vi "ODMR sweep set MW control.vi"(8 "Save?":bool, 9 "file path (dialog if empty)":path=path "C:/Users/Ouyang Group/Documents/Data/5-13-15/ND Au 686 ODMR sweep 1", 10 "Freq Sweep Cluster":T1={"GPIB address 2"="19", "resolution (10 Hz:2) 2"=2, "band (1-26.5:2) 2"=2, "Freq max"=3300000000.0, "Start Freq"=5.5, "freq Step"=0.02, "rate"=100.0, "samples per channel"=500} {"rate" format="%0.2f"; "resolution (10 Hz:2) 2" items=["0.1 Hz", "1 Hz", "10 Hz", "100 Hz", "1 KHz", "10 KHz", "100 KHz", "1 MHz", "10 MHz", "100 MHz", "1 GHz"]}, 11 "Dot Tracking Cluster":T2={"RS232 settings"={"Portnumber"=6, "Baudrate"=5}, "X Parameters"={"Number of X Steps"=200, "Max X (V)"=2.0, "Min X (V)"=-2.0}, "Y Parameters"={"Number of Y Steps"=200, "Max Y (V)"=2.0, "Min Y (V)"=-2.0}, "X Pos"=97.0, "Y Pos"=112.0, "Z Pos"=52.78, "Tracking interval"=150.0} {"RS232 settings"."Portnumber" items=["COM1", "COM2", "COM3", "COM4", "COM5", "COM6", "COM7", "COM8", "COM9", "COM10", "COM11", "COM12", "COM13", "COM14", "COM15", "COM16", "COM17", "COM18", "COM19", "COM20", "COM21", "COM22", "COM23", "COM24", "COM25", "COM26", "COM27", "COM28", "COM29", "COM30"]; "RS232 settings"."Baudrate" items=["9600", "14400", "19200", "38400", "57600", "115200"]}) -> (0 "Z Position":dbl=31.0, 1 "Y Position":dbl=62.0, 2 "X Position":dbl=97.0, 3 "XY Graph":cluster{"Y":dbl[], "Y":dbl[]}[](graph), 4 "appended array":ext[][](array[numeric]))   [LabVIEW 2012]
uses:
  <vilib>/DAQmx/read.llb/DAQmx Read (Counter 1D DBL 1Chan NSamp).vi
  <vilib>/DAQmx/create/channels.llb/DAQmx Create Channel (CI-Count Edges).vi
  <vilib>/DAQmx/configure/timing.llb/DAQmx Timing (Sample Clock).vi
  <vilib>/DAQmx/miscellaneous.llb/DAQmx Fill In Error Info.vi
  <vilib>/Utility/file.llb/Write To Spreadsheet File (DBL).vi
  <resource>/objmgr/daqmx.rc
panel:
  out "power compensated":ext
  out "freq":dbl
  in  "stop":bool
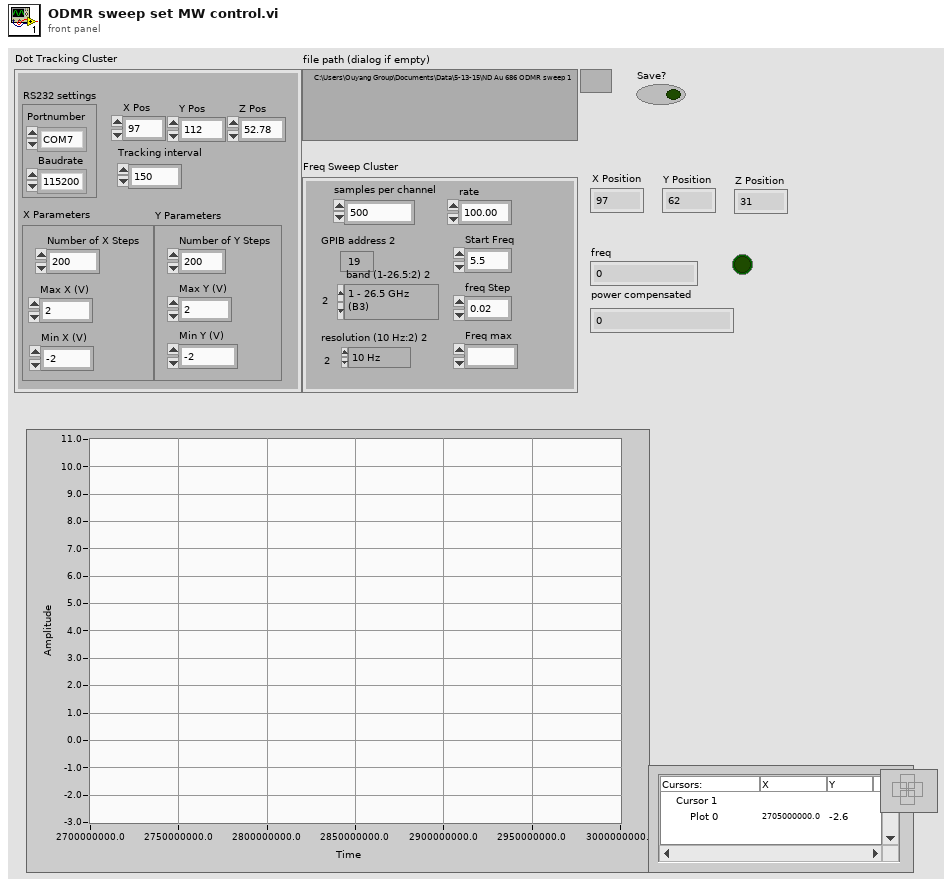
[diagram p1: front panel]
types:
  T1 = cluster{"GPIB address 2":string, "resolution (10 Hz:2) 2":i32, "band (1-26.5:2) 2":i32, "Freq max":ext, "Start Freq":dbl, "freq Step":dbl, "rate":dbl, "samples per channel":i32}
  T2 = cluster{"RS232 settings":cluster{"Portnumber":i32, "Baudrate":u16}, "X Parameters":cluster{"Number of X Steps":i32, "Max X (V)":dbl, "Min X (V)":dbl}, "Y Parameters":cluster{"Number of Y Steps":i32, "Max Y (V)":dbl, "Min Y (V)":dbl}, "X Pos":dbl, "Y Pos":dbl, "Z Pos":dbl, "Tracking interval":dbl}
  T3 = cluster{"Number of X Steps":i32, "Max X (V)":dbl, "Min X (V)":dbl}
  T4 = cluster{"Number of Y Steps":i32, "Max Y (V)":dbl, "Min Y (V)":dbl}
  T5 = cluster{"source lock":bool, "lock frequency (Hz)":ext, "coarse tune":bool}
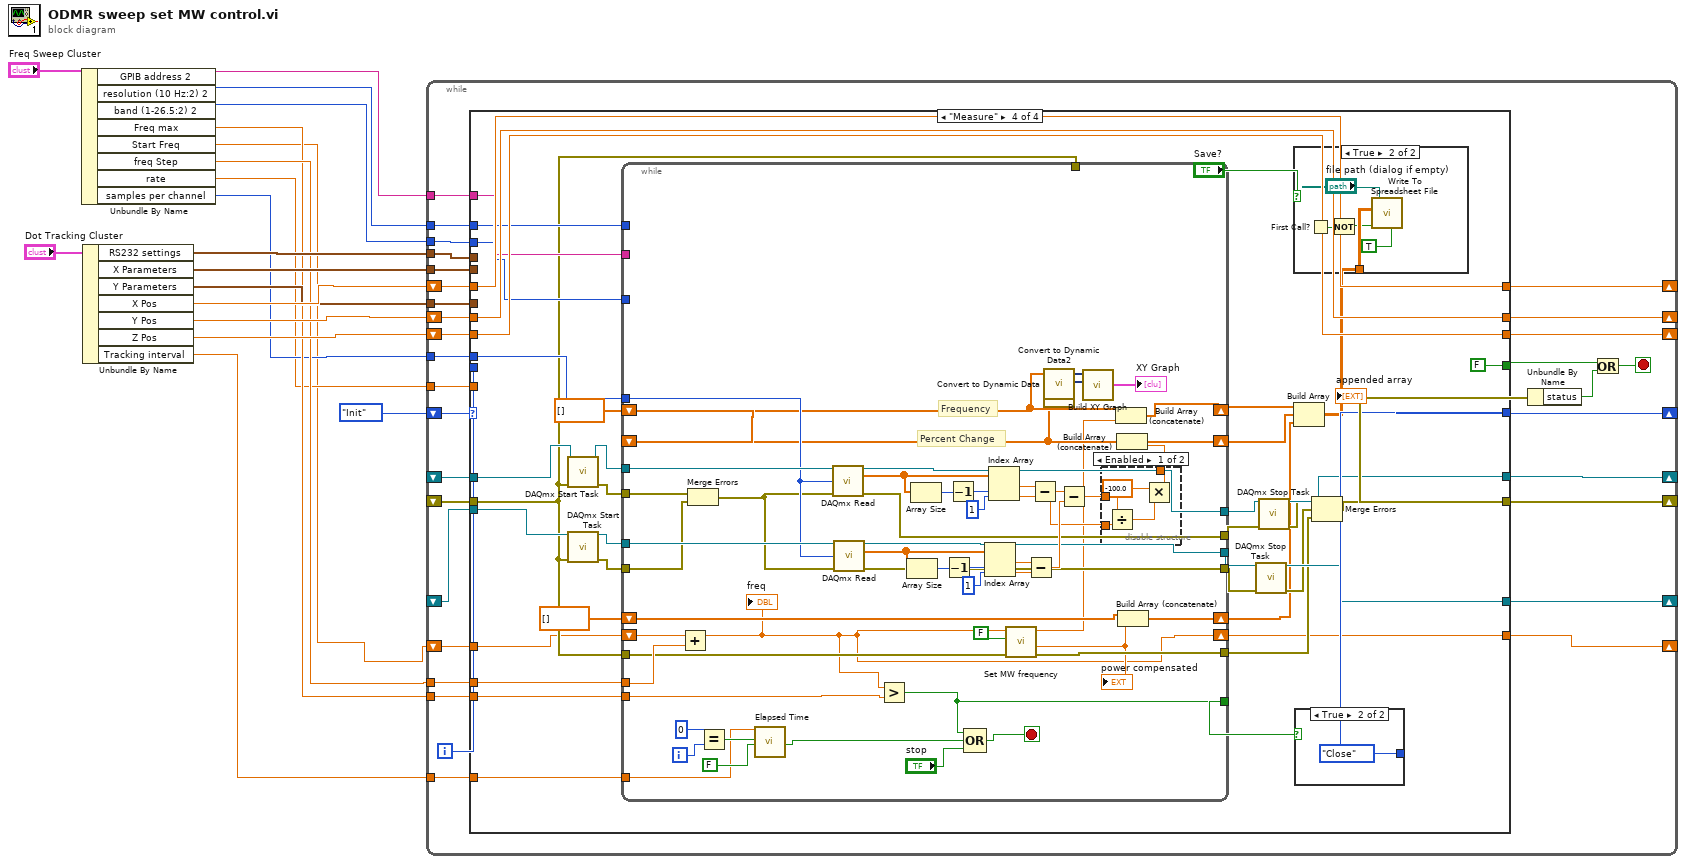
[diagram p0: block diagram]
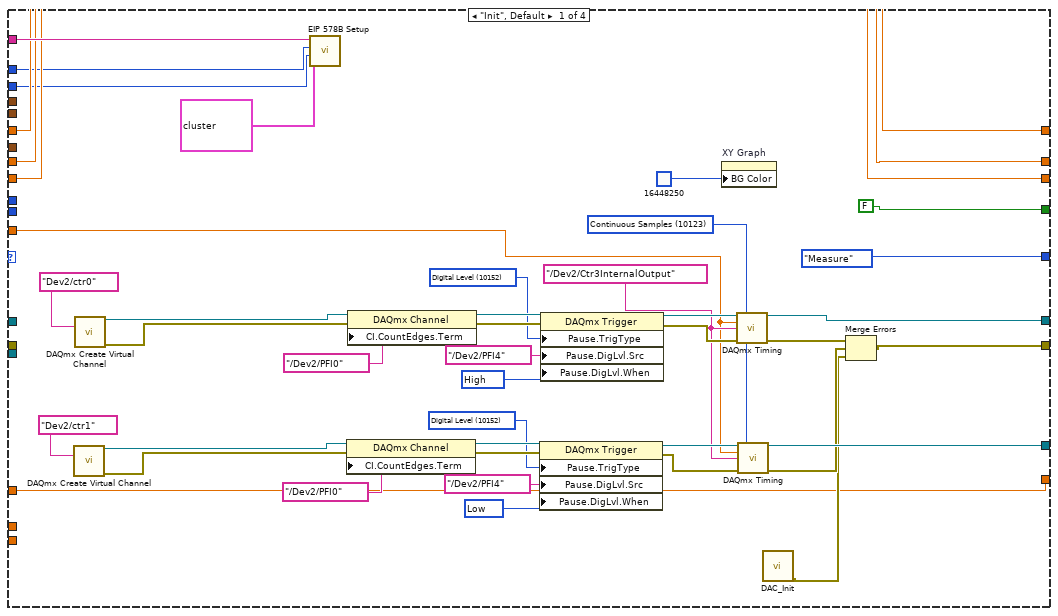
[diagram p2: hidden frame]
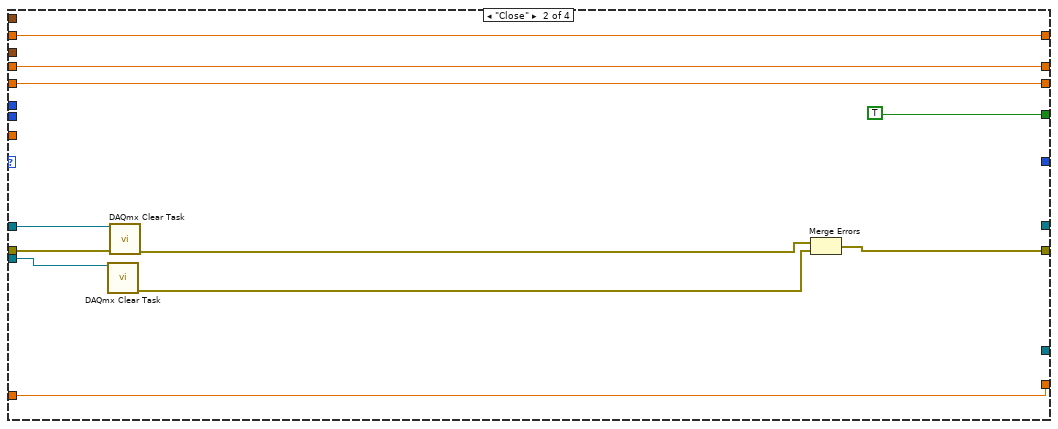
[diagram p3: hidden frame]
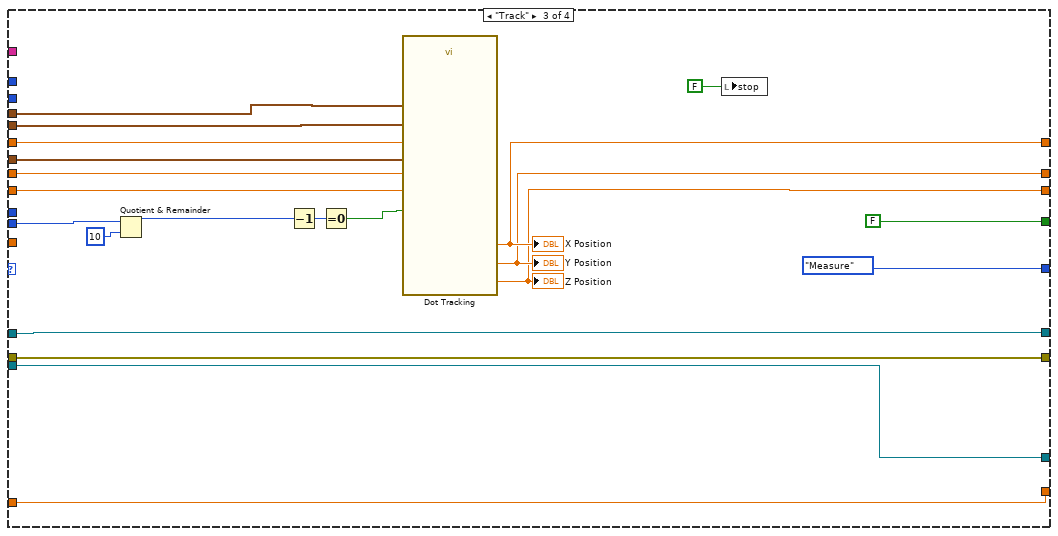
[diagram p4: hidden frame]
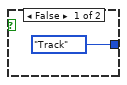
[diagram p6: hidden frame]
diagram:
  n1 = Unbundle By Name("Freq Sweep Cluster") -> ("GPIB address 2"=w8:string, "resolution (10 Hz:2) 2"=w7:i32, "band (1-26.5:2) 2"=w6:i32, "Freq max"=w4:ext, "Start Freq"=w1:dbl, "freq Step"=w5:dbl, "rate"=w2:dbl, "samples per channel"=w3:i32)
  n2 = Unbundle By Name("Dot Tracking Cluster") -> ("RS232 settings"=w13:cluster{"Portnumber":i32, "Baudrate":u16}, "X Parameters"=w12:T3, "Y Parameters"=w11:T4, "X Pos"=w16:dbl, "Y Pos"=w15:dbl, "Z Pos"=w14:dbl, "Tracking interval"=w10:dbl)
  n3 = while {
    shift-right: [w45] -> _
    shift-left: enum16{"Init", "Measure", "Track", "Close"}."Init" -> [w49]
    tunnel: w8 -> [w48]
    shift-right: [w47] -> _
    shift-left: _ -> [w44]
    shift-right: [w46] -> _
    shift-left: _ -> [w43]
    shift-right: [w40] -> _
    shift-left: _ -> [w42]
    tunnel: w3 -> [w37]
    shift-right: [w32] -> _
    shift-left: w16 -> [w35]
    shift-right: [w31] -> _
    shift-left: w15 -> [w34]
    shift-right: [w30] -> _
    shift-left: w14 -> [w33]
    tunnel: w7 -> [w29]
    tunnel: w6 -> [w28]
    shift-right: [w25] -> _
    shift-left: w1 -> [w27]
    tunnel: w5 -> [w26]
    tunnel: w13 -> [w24]
    tunnel: w12 -> [w23]
    tunnel: w11 -> [w22]
    tunnel: w10 -> [w21]
    tunnel: w4 -> [w20]
    tunnel: w2 -> [w19]
    i -> [w41]
    stop <- w39 stop-if-true
    n4 = case shown="\"Measure\"" w49 {
      tunnel: [FALSE TRUE FALSE FALSE] -> w38
      tunnel: w48 -> [w90 _ _ w142]
      tunnel: [w65 _ w123 w152] -> w47
      tunnel: [w64 _ w122 w149] -> w46
      tunnel: [w61 w97 w116 w162] -> w40
      tunnel: [enum16{"Init", "Measure", "Track", "Close"}."Measure" _ enum16{"Init", "Measure", "Track", "Close"}."Measure" w161] -> w45
      tunnel: w44 -> [_ w101 w123 w158]
      tunnel: w43 -> [_ w99 w122 w155]
      tunnel: w42 -> [_ w100 w116 w137]
      tunnel: w41 -> [_ _ w117 _]
      tunnel: w37 -> [_ _ _ w147]
      tunnel: w35 -> [w57 w95 w112 w145]
      tunnel: w34 -> [w56 w94 w111 w144]
      tunnel: w33 -> [w55 w93 w110 w143]
      tunnel: [w57 w95 w109 w145] -> w32
      tunnel: [w56 w94 w108 w144] -> w31
      tunnel: [w55 w93 w107 w143] -> w30
      tunnel: w29 -> [w54 _ _ w141]
      tunnel: w28 -> [w53 _ _ w140]
      tunnel: w27 -> [w51 w92 w106 w135]
      tunnel: w26 -> [_ _ _ w134]
      tunnel: [w51 w92 w106 w133] -> w25
      tunnel: w24 -> [_ _ w105 _]
      tunnel: w23 -> [_ _ w104 _]
      tunnel: w22 -> [_ _ w103 _]
      tunnel: w21 -> [_ _ _ w132]
      tunnel: w20 -> [_ _ _ w131]
      tunnel: w19 -> [w50 _ _ _]
      frame "Init", Default {
        w66 = tag "/Dev2/Ctr3InternalOutput" ("source")
        w67 = 10123 items=["Finite Samples"=10178, "Continuous Samples"=10123, "Hardware Timed Single Point"=12522] ("sample mode")
        w72 = 10214 items=["High"=10192, "Low"=10214] ("Pause.DigLvl.When")
        w74 = 10152 items=["Analog Level"=10101, "Analog Window"=10103, "Digital Level"=10152, "Digital Pattern"=10398, "None"=10230] ("Pause.TrigType")
        w81 = 10192 items=["High"=10192, "Low"=10214] ("Pause.DigLvl.When")
        w83 = 10152 items=["Analog Level"=10101, "Analog Window"=10103, "Digital Level"=10152, "Digital Pattern"=10398, "None"=10230] ("Pause.TrigType")
        n5 = call-poly <vilib>:"DAQmx Create Virtual Channel.vi"("counter"=tag "Dev2/ctr1") -> ("task out"=w79:refnum<k21>, "error out"=w78:errorcluster)  [unwired: 13 in]
        n6 = call-poly <vilib>:"DAQmx Create Virtual Channel.vi"("counter"=tag "Dev2/ctr0") -> ("task out"=w88:refnum<k21>, "error out"=w87:errorcluster)  [unwired: 13 in]
        n7 = call "EIP 578B Setup.vi"("GPIB Address"=w90, "band (1-26.5 GHz:20)"=w54, "resolution (1 Hz:1)"=w53, "source locking"=T5 {"source lock"=FALSE, "lock frequency (Hz)"=1000000000.0, "coarse tune"=TRUE}) -> ()  [unwired: 2 in, 2 out]
        n8 = property class="DAQmx Channel"(reference=w79, error in=w78, "CI.CountEdges.Term"=tag "/Dev2/PFI0") -> (reference out=w76:refnum<k21>, error out=w75:errorcluster)
        n9 = property class="DAQmx Channel"(reference=w88, error in=w87, "CI.CountEdges.Term"=tag "/Dev2/PFI0") -> (reference out=w85:refnum<k21>, error out=w84:errorcluster)
        n10 = property class="DAQmx Trigger"(reference=w76, error in=w75, "Pause.TrigType"=w74, "Pause.DigLvl.Src"=tag "/Dev2/PFI4", "Pause.DigLvl.When"=w72) -> (reference out=w69:refnum<k21>, error out=w68:errorcluster)
        n11 = property class="DAQmx Trigger"(reference=w85, error in=w84, "Pause.TrigType"=w83, "Pause.DigLvl.Src"=tag "/Dev2/PFI4", "Pause.DigLvl.When"=w81) -> (reference out=w71:refnum<k21>, error out=w70:errorcluster)
        n12 = property on="XY Graph" class="XYGraph (strict)"("BG Color"=u32 16448250) -> ()  [unwired: 2 in, 2 out]
        n13 = call-poly <vilib>:"DAQmx Timing.vi"("task/channels in"=w71, "sample mode"=w67, "rate"=w50, "source"=w66, "error in"=w70) -> ("task out"=w65:refnum<k21>, "error out"=w63:errorcluster)  [unwired: 9 in]
        n14 = call-poly <vilib>:"DAQmx Timing.vi"("task/channels in"=w69, "sample mode"=w67, "rate"=w50, "source"=w66, "error in"=w68) -> ("task out"=w64:refnum<k21>, "error out"=w62:errorcluster)  [unwired: 9 in]
        n15 = call "DAC_Init.vi"() -> ("error out"=w52:errorcluster)  [unwired: 11 in]
        n16 = Merge Errors(w63, w62, w52) -> (w61:errorcluster)
      }
      frame "Close" {
        n17 = call <vilib>:"DAQmx Clear Task.vi"("task in"=w99) -> ("error out"=w98:errorcluster)  [unwired: 14 in]
        n18 = call <vilib>:"DAQmx Clear Task.vi"("task in"=w101, "error in"=w100) -> ("error out"=w96:errorcluster)  [unwired: 13 in]
        n19 = Merge Errors(w96, w98) -> (w97:errorcluster)
      }
      frame "Track" {
        n20 = Quotient & Remainder(x=w117, y=10) -> (x-y*floor(x/y)=w120:i32)  [unwired: 1 out]
        n21 = Decrement(x=w120) -> (x-1=w121:i32)
        n22 = Equal To 0?(x=w121) -> (x = 0?=w118:bool)
        n23 = call "Dot Tracking.vi"("X"=w104, "Y Parameters"=w103, "RS232 settings"=w105, "X Pos"=w112, "Y pos"=w111, "Z Pos"=w110, "Z-track?"=w118) -> ("X Position"=w109:dbl, "Y Position"=w108:dbl, "Z Position"=w107:dbl)  [unwired: 2 in, 4 out]
        "X Position" <- w109
        "Y Position" <- w108
        "Z Position" <- w107
        n24 = local write "stop"(FALSE ("stop")) -> ()
      }
      frame "Measure" {
        w146 = dbl[] []
        n25 = call <vilib>:"DAQmx Start Task.vi"("task/channels in"=w158, "error in"=w137) -> ("task out"=w156:refnum<k21>, "error out"=w157:errorcluster)  [unwired: 12 in]
        n26 = call <vilib>:"DAQmx Start Task.vi"("task/channels in"=w155, "error in"=w137) -> ("task out"=w154:refnum<k21>, "error out"=w153:errorcluster)  [unwired: 12 in]
        n27 = while {
          shift-right: [w208] -> w126
          shift-left: w146 -> [w195]
          shift-right: [w207] -> w127
          shift-left: w146 -> [w197]
          tunnel: w154 -> [w204]
          tunnel: [w203] -> w151
          tunnel: [w202] -> w160
          tunnel: [w199] -> w159
          tunnel: w157 -> [w201]
          tunnel: w156 -> [w200]
          tunnel: w153 -> [w184]
          tunnel: w147 -> [w198]
          tunnel: w142 -> [_]
          tunnel: w141 -> [_]
          tunnel: w140 -> [_]
          tunnel: w137 -> [_]
          tunnel: [w182] -> w139
          tunnel: [w181] -> w138
          tunnel: w137 -> [w174]
          tunnel: [w174] -> w136
          shift-right: [w171] -> w133
          shift-left: w135 -> [w180]
          tunnel: w134 -> [w179]
          tunnel: w132 -> [w178]
          tunnel: w131 -> [w177]
          shift-right: [w176] -> w125
          shift-left: dbl[] [] -> [w175]
          i -> [w189]
          stop <- w185 stop-if-true
          # "Percent Change"
          # "Frequency"
          n28 = Add(x=w180, y=w179) -> (x+y=w171:dbl)
          "freq" <- w171
          n29 = Merge Errors(w201, w184) -> (w183:errorcluster)
          n30 = Equal?(x=0, y=w189) -> (x = y?=w188:bool)
          n31 = call "Elapsed Time"("Time Target (s)"=w178, "Reset"=w188, "Auto Reset"=FALSE) -> ("Time has Elapsed"=w187:bool)  [unwired: 9 in, 7 out]
          n32 = call-poly <vilib>:"DAQmx Read.vi"("task/channels in"=w200, "number of samples per channel"=w198, "error in"=w183) -> ("task out"=w202:refnum<k21>, "data"=w221:dbl[], "error out"=w203:errorcluster)  [unwired: 10 in]
          n33 = call-poly <vilib>:"DAQmx Read.vi"("task/channels in"=w204, "number of samples per channel"=w198, "error in"=w183) -> ("task out"=w199:refnum<k21>, "data"=w210:dbl[], "error out"=w181:errorcluster)  [unwired: 10 in]
          n34 = Greater?(x=w171, y=w177) -> (0:w182:bool)
          n35 = Array Size(array=w210) -> (size(s)=w215:i32)
          n36 = Array Size(array=w221) -> (size(s)=w220:i32)
          n37 = Decrement(x=w215) -> (x-1=w214:i32)
          n38 = Decrement(x=w220) -> (x-1=w219:i32)
          n39 = Compound Arithmetic op=OR(w182, w187, "stop") -> (w185:bool)
          n40 = Index Array(array=w210, index #1=w214, index #2=1 ("index")) -> (element #1=w211:dbl, element #2=w212:dbl)
          n41 = Index Array(array=w221, index #1=w219, index #2=1 ("index")) -> (element #1=w216:dbl, element #2=w217:dbl)
          n42 = call "Set MW frequency.vi"("source lock"=FALSE, "freq"=w171) -> ("power compensated"=w172:ext, "frequency (Hz)"=w170:ext)  [unwired: 7 in, 1 out]
          "power compensated" <- w172
          n43 = Subtract(x=w211, y=w212) -> (x-y=w209:dbl)
          n44 = Subtract(x=w216, y=w217) -> (x-y=w205:dbl)
          n45 = call "Convert to Dynamic Data"("Array"=w197) -> ("Dynamic Data Type"=w196:dynamicdata)  [unwired: 3 in]
          n46 = call "Convert to Dynamic Data2"("Array"=w195) -> ("Dynamic Data Type"=w194:dynamicdata)  [unwired: 3 in]
          n47 = Subtract(x=w205, y=w209) -> (x-y=w206:dbl)
          n48 = call "Build XY Graph"("Y Input"=w194, "X Input"=w196) -> ("XY Graph"=→"XY Graph":cluster{"Y":dbl[], "Y":dbl[]}[])  [unwired: 3 in, 6 out]
          n49 = disable-structure shown="Enabled" {
            disable-tunnel: w206 -> [w226 w227]
            disable-tunnel: w205 -> [w225 _]
            disable-tunnel: [w223 w227] -> w192
            frame Enabled {
              n50 = Divide(x=w226, y=w225) -> (x/y=w224:dbl)
              n51 = Multiply(x=-100.0, y=w224) -> (x*y=w223:dbl)
            }
            frame Disabled {
            }
          }
          n52 = Build Array (concatenate)(w197, w170) -> (w207:ext[])
          n53 = Build Array (concatenate)(w195, w192) -> (w208:dbl[])
          n54 = Build Array (concatenate)(w175, w172) -> (w176:ext[])
        }
        n55 = call <vilib>:"DAQmx Stop Task.vi"("task/channels in"=w159, "error in"=w138) -> ("task out"=w149:refnum<k21>, "error out"=w148:errorcluster)  [unwired: 12 in]
        n56 = call <vilib>:"DAQmx Stop Task.vi"("task/channels in"=w160, "error in"=w151) -> ("task out"=w152:refnum<k21>, "error out"=w150:errorcluster)  [unwired: 12 in]
        n57 = Build Array(w127, w126, w125) -> (w124:ext[][])
        "appended array" <- w124
        n58 = case shown="True" "Save?" {
          tunnel: w124 -> [_ w167]
          frame False {
          }
          frame True {
            n59 = First Call?() -> (First Call?: T/F=w166:bool)
            n60 = Not(x=w166) -> (.not. x?=w165:bool)
            n61 = call-poly <vilib>:"Write To Spreadsheet File.vi"("transpose? (no:F)"=TRUE, "append to file? (new file:F)"=w165, "2D data"=w167, "file path (dialog if empty)"="file path (dialog if empty)") -> ()  [unwired: 4 in, 1 out]
          }
        }
        n62 = case shown="True" w139 {
          tunnel: [enum16{"Init", "Measure", "Track", "Close"}."Track" enum16{"Init", "Measure", "Track", "Close"}."Close"] -> w161
          frame False {
          }
          frame True {
          }
        }
        n63 = Merge Errors(w150, w148, w136) -> (w162:errorcluster)
      }
    }
    n64 = Unbundle By Name(w40) -> ("status"=w36:bool)
    n65 = Or(x=w38, y=w36) -> (x .or. y?=w39:bool)
  }
